vi "RTS Client Analysis.vi"(8 "Error In":errorcluster) -> (0 "Error Out":errorcluster)   [LabVIEW 2016]
uses:
  <vilib>/Utility/file.llb/Read Delimited Spreadsheet (string).vi
panel:
  out "Organized File Open List":path[](array[path])
  out "Full Data List":path[](array[path])
  out "1D String":string[][](array[string])
  in  "OldVal":i32[](array[numeric])
  out "Mixed Signal Graph 2":T1(graph)
  out "Headers":string[](array[string])
  out "Initial Headers":string[][](array[string])
  in  "File Location":path
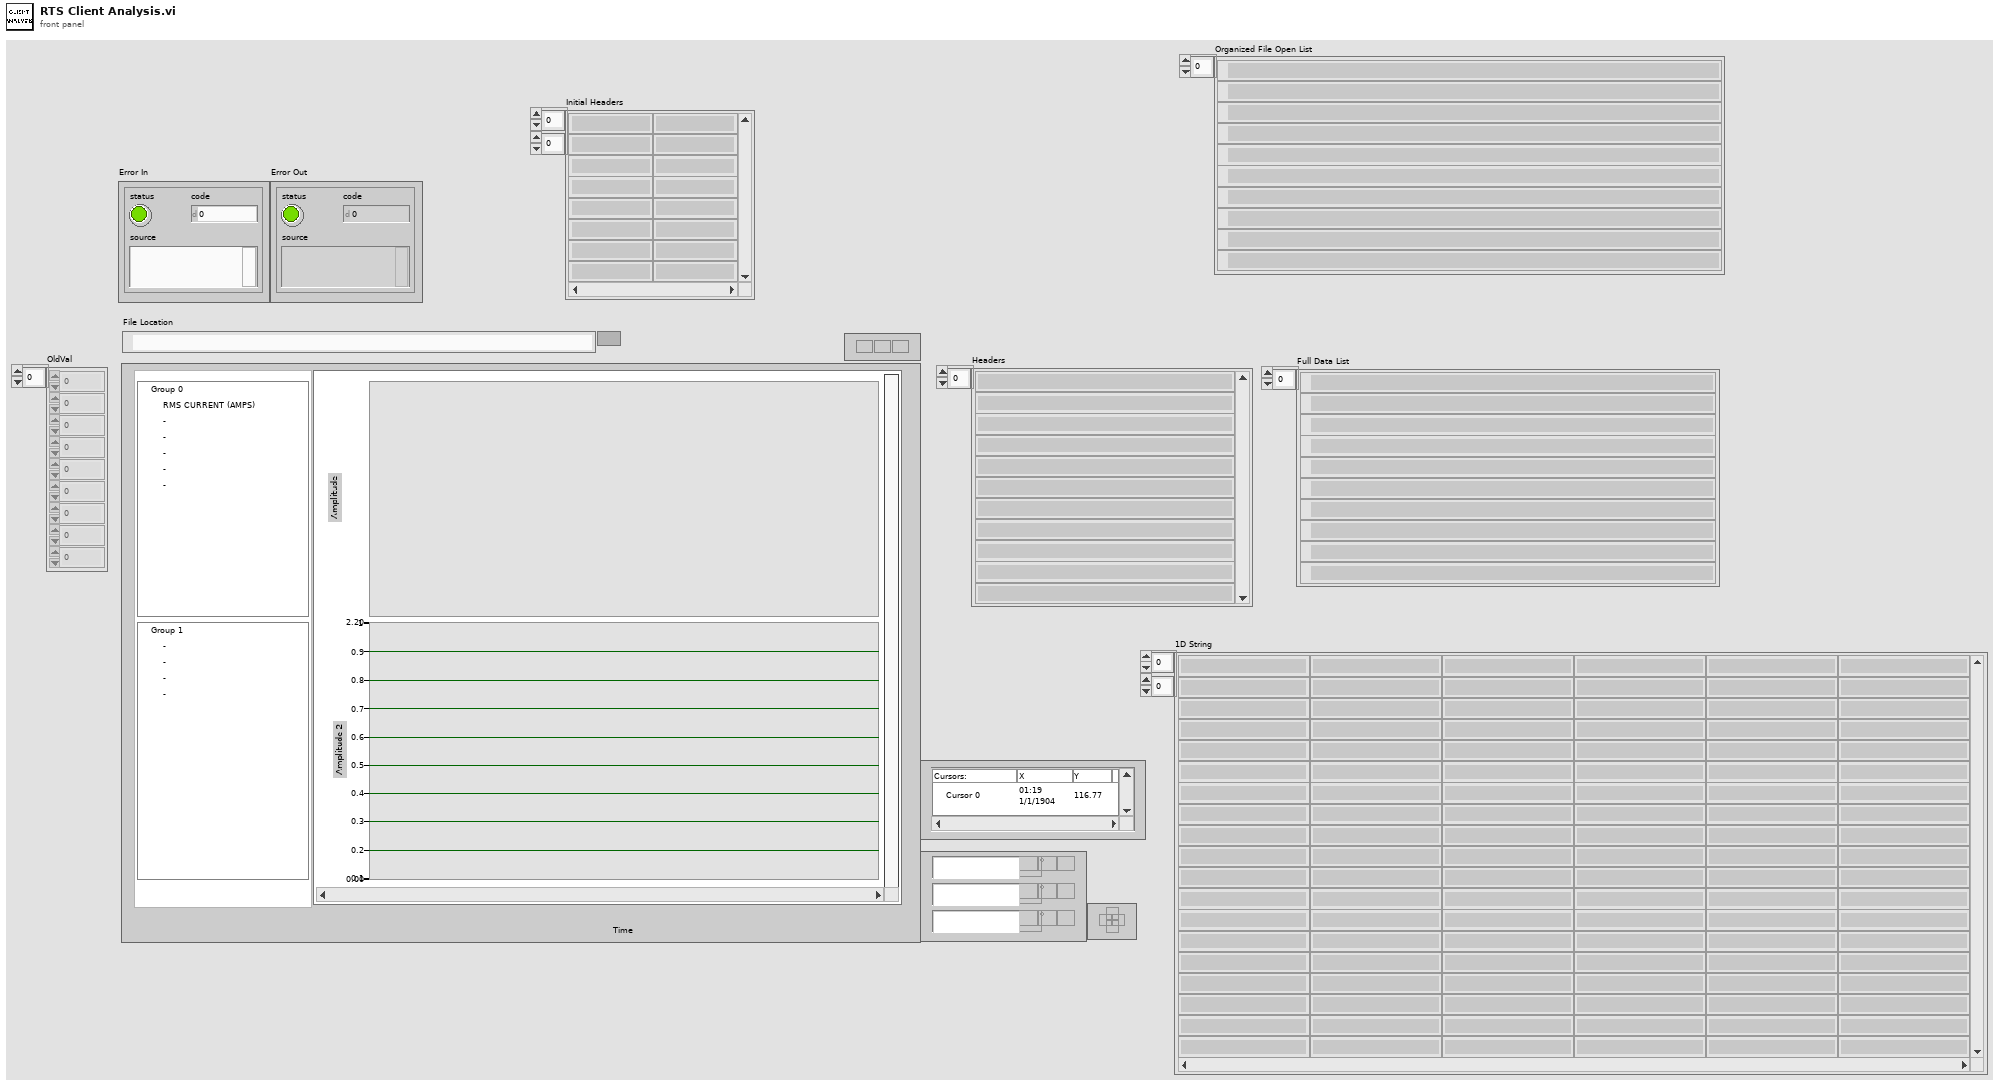
[diagram p1: front panel]
types:
  T1 = cluster{"Waveform Graph":waveform(dbl), "Waveform Graph":waveform(dbl), "Waveform Graph":waveform(dbl), "Waveform Graph":waveform(dbl), "Waveform Graph":waveform(dbl), "Waveform Graph":waveform(dbl), "Waveform Graph":waveform(dbl), "Waveform Graph":waveform(dbl), "Waveform Graph":waveform(dbl), "Waveform Graph":waveform(dbl)}
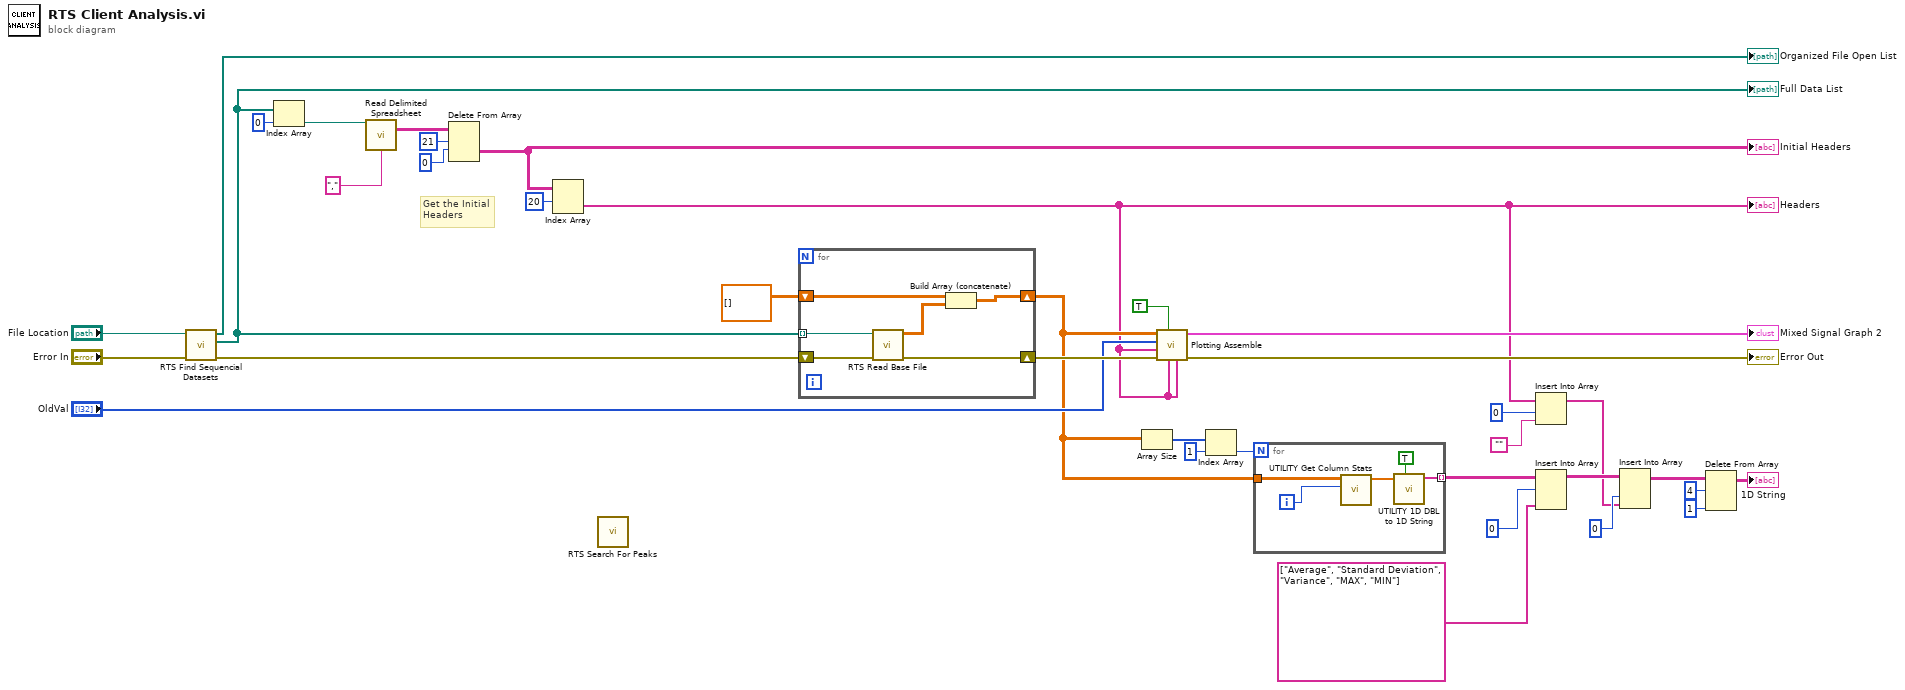
[diagram p0: block diagram]
diagram:
  # "Get the Initial\nHeaders"
  n1 = call "RTS Find Sequencial Datasets.vi"("Error In"="Error In", "File Location"="File Location") -> ("Error Out"=w34:errorcluster, "Full Data List"=w28:path[], "Organized File Open List"=→"Organized File Open List":path[])  [unwired: 7 in]
  "Full Data List" <- w28
  n2 = Index Array(array=w28, index=0) -> (element=w26:path)
  n3 = call-poly <vilib>:"Read Delimited Spreadsheet.vi"("file path (dialog if empty)"=w26, "delimiter (\\t)"="," ("delimiter (\\t)")) -> ("all rows"=w31:string[][])  [unwired: 8 in, 5 out]
  n4 = Delete From Array(array=w31, length=21, index (row)=0 ("disabled index (col)")) -> (deleted portion=w25:string[][])  [unwired: 1 in, 1 out]
  "Initial Headers" <- w25
  n5 = Index Array(array=w25, index (row)=20) -> (element=w9:string[])  [unwired: 1 in]
  "Headers" <- w9
  n6 = call "RTS Search For Peaks.vi"() -> ()  [unwired: 12 in]
  n7 = for {
    tunnel: w28 -> [w42] mode=indexing
    shift-right: [w40] -> w22
    shift-left: w34 -> [w41]
    shift-right: [w38] -> w18
    shift-left: dbl[][] [] -> [w39]
    n8 = call "RTS Read Base File.vi"("Error In"=w41, "File Location"=w42) -> ("Error Out"=w40:errorcluster, "all rows"=w37:dbl[][])  [unwired: 8 in]
    n9 = Build Array (concatenate)(w39, w37) -> (w38:dbl[][])
  }
  n10 = Array Size(array=w18) -> (size(s)=w17:i32[])
  n11 = call "Plotting Assemble.vi"("Custom Titles"=w9, "Listbox Item Names"=w9, "Use Filter?"=TRUE, "Error In"=w22, "Full Item Names"=w9, "OldVal"="OldVal", "All Data"=w18) -> ("Error Out"=→"Error Out":errorcluster, "Mixed Signal Graph"=→"Mixed Signal Graph 2":T1)  [unwired: 3 in]
  n12 = Index Array(array=w17, index=1) -> (element=w15:i32)
  n13 = for {
    N: w15 -> [_]
    tunnel: w18 -> [w47]
    tunnel: [w43] -> w14 mode=indexing
    i -> [w46]
    n14 = call "UTILITY Get Column Stats.vi"("Index"=w46, "Draw Stats"=w47) -> ("Column Stats"=w45:dbl[])  [unwired: 8 in, 1 out]
    n15 = call "UTILITY 1D DBL to 1D String.vi"("DBL?"=TRUE, "1D DBL"=w45) -> ("1D String"=w43:string[])  [unwired: 9 in]
  }
  n16 = Insert Into Array(array=w9, index=0, new element="") -> (w6:string[])
  n17 = Insert Into Array(array=w14, index (row)=0, new element=string[] ["Average", "Standard Deviation", "Variance", "MAX", "MIN"]) -> (w11:string[][])  [unwired: 1 in]
  n18 = Insert Into Array(array=w11, index (col)=0 ("index (row)"), new element=w6) -> (w5:string[][])  [unwired: 1 in]
  n19 = Delete From Array(array=w5, length=4, index (row)=1) -> (array with subset deleted=→"1D String":string[][])  [unwired: 1 in, 1 out]
